vi "Create All Custom Chars.vi"(8 "error in (no error)":errorcluster, 9 "All Chars":T2, 10 "VISA resource name in":refnum<visa-resource-name>, 11 "LCD-I2C in":refnum<class "LCD-I2C.lvclass">) -> (0 "error out":errorcluster, 2 "VISA resource name":refnum<visa-resource-name>, 3 "LCD-I2C out":refnum<class "LCD-I2C.lvclass">)   [LabVIEW 2023, in "CTI-Visa-DeviceLib.lvlib" / "LCD-I2C.lvclass"]
uses:
  LCD-I2C.lvclass
  Custom Char.ctl
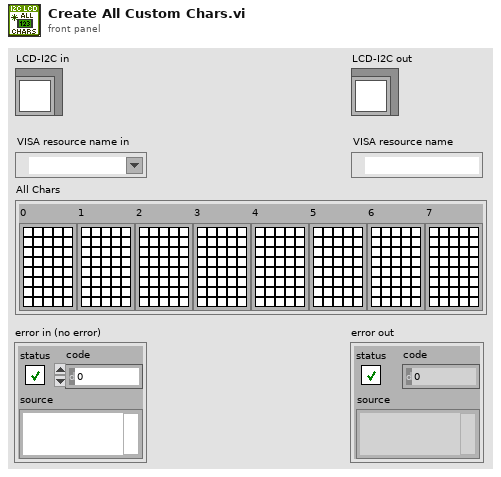
[diagram p1: front panel]
types:
  T1 = typedef "CTI-Visa-DeviceLib.lvlib/LCD-I2C.lvclass/Custom Char.ctl" = bool[][]
  T2 = cluster{"0":T1, "1":T1, "2":T1, "3":T1, "4":T1, "5":T1, "6":T1, "7":T1}
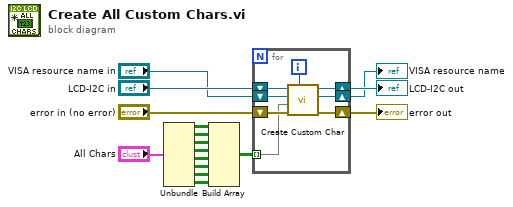
[diagram p0: block diagram]
diagram:
  n1 = Unbundle("All Chars") -> ("0"=w15:T1, "1"=w8:T1, "2"=w9:T1, "3"=w10:T1, "4"=w11:T1, "5"=w12:T1, "6"=w13:T1, "7"=w14:T1)
  n2 = Build Array(w15, w8, w9, w10, w11, w12, w13, w14) -> (w7:bool[][][])
  n3 = for {
    tunnel: w7 -> [w17] mode=indexing
    shift-right: [w18] -> w3
    shift-left: "error in (no error)" -> [w23]
    shift-right: [w19] -> w2
    shift-left: "LCD-I2C in" -> [w24]
    shift-right: [w20] -> w1
    shift-left: "VISA resource name in" -> [w21]
    i -> [w22]
    n4 = call "Create Custom Char.vi"("Location 0-7"=w22, "error in (no error)"=w23, "Char"=w17, "VISA resource name in"=w21, "LCD-I2C in"=w24) -> ("error out"=w18:errorcluster, "VISA resource name"=w20:refnum<visa-resource-name>, "LCD-I2C out"=w19:refnum<class "LCD-I2C.lvclass">)  [unwired: 4 in]
  }
  "error out" <- w3
  "LCD-I2C out" <- w2
  "VISA resource name" <- w1
